vi "Handle Error.vi"(7 "Stop on Unhandled Error (T)":bool=TRUE, 8 "error in":errorcluster, 11 "MeasuringDevice":refnum<class "MeasuringDevice.lvclass">) -> (0 "handling error":errorcluster, 2 "Unhandled error":errorcluster, 3 "MeasuringDevice out":refnum<class "MeasuringDevice.lvclass">)   [LabVIEW 2017, in "MeasuringDevice.lvclass"]
doc: "JKI State Machine Objects (SMO) 1.0.0.11\nJKI - JKI\nCopyright (c) 2016, JKIJKI State Machine Objects (SMO) 1.3.0.56\nJKI - JKI\nCopyright (c) 2017, JKI"
uses:
  MeasuringDevice.lvclass
  Device/Device.lvclass
panel:
  # "For instructions on how to use the JKI State Machine Objects, examples and video tutorials, visit:\nhttp://jki.net/state-machine-objects/\n\nJKI State Machine Objects™\nhttp://jki.net/state-machine-objects/\nCopyright (C) 2005-2015, JKI <info@jki.net>\nALL RIGHTS RESERVED"
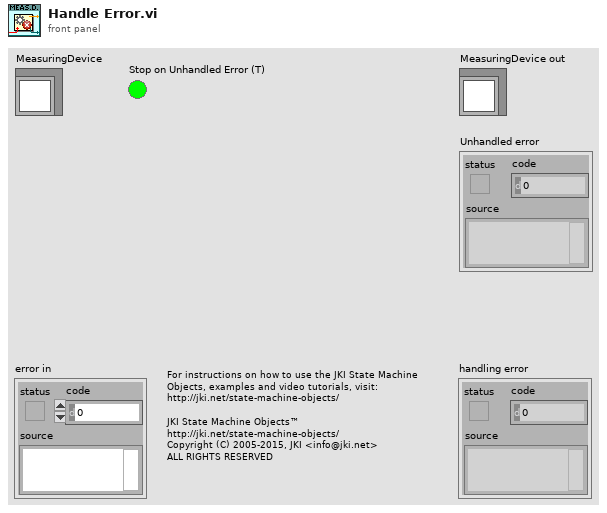
[diagram p1: front panel]
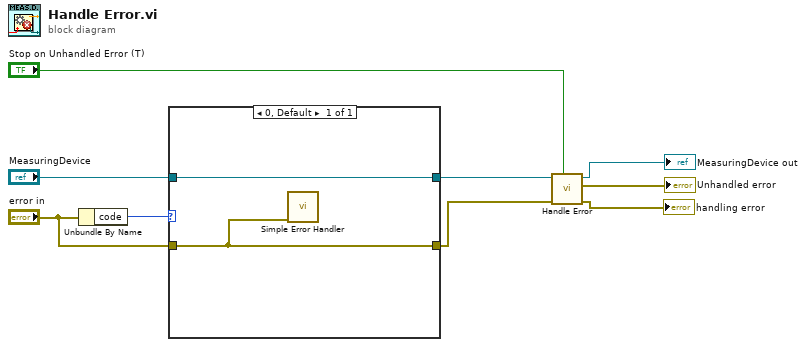
[diagram p0: block diagram]
diagram:
  n1 = Unbundle By Name("error in") -> ("code"=w6:i32)
  n2 = case shown="0, Default" w6 {
    tunnel: "MeasuringDevice" -> [w11]
    tunnel: "error in" -> [w10]
    tunnel: [w11] -> w3
    tunnel: [w10] -> w1
    frame 0, Default {
      n3 = call <vilib>:"Simple Error Handler.vi"("error in (no error)"=w10) -> ()  [unwired: 4 in, 5 out]
    }
  }
  n4 = call-parent "Handle Error.vi"("Stop on Unhandled Error (T)"="Stop on Unhandled Error (T)", "error in"=w1, "SMO"=w3) -> ("handling error"=→"handling error":errorcluster, "Unhandled error"=→"Unhandled error":errorcluster, "SMO out"=→"MeasuringDevice out":refnum<class "MeasuringDevice.lvclass">)  [unwired: 6 in]
